vi "Dig.vi"(8 "Error In":errorcluster, 10 "Selection List[]":refnum<vi>[](array[refnum]), 11 "VI In":refnum<vi>) -> (0 "Error Out":errorcluster, 3 "VI Out":refnum<vi>)   [LabVIEW 2017, in "Toolkit VIs.lvlib"]
doc: "A VI script that encloses a selection of code in a Diagram Disable Contional structure, creates a duplicate of the original code to be refactored for the Enabled frame, adds an \"Original\" and \"Refactored\" subdiagram label to each frame, respectively, and adds a bookmark with \"RIP\", the DoD (Date of Death), and grave digger (programmer) as the structure's label.\n\nBy default, today's date is used as the DoD and the application's user name is used for the grave digger."
uses:
  Toolkit VIs.lvlib
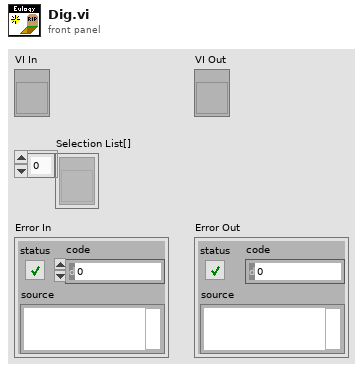
[diagram p1: front panel]
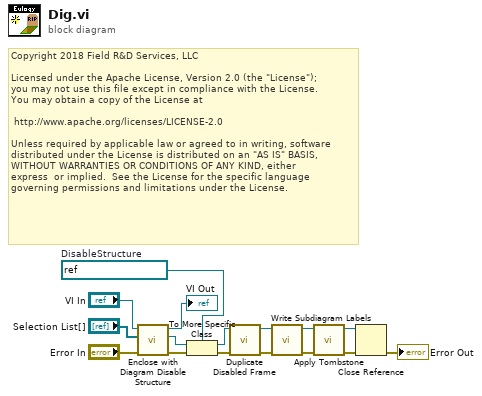
[diagram p0: block diagram]
diagram:
  w15 = refnum<vi> refnum  # DisableStructure
  # "Copyright 2018 Field R&D Services, LLC\n\nLicensed under the Apache License, Version 2.0 (the \"License\");\nyou may not use this file except in compliance with the License.\nYou may obtain a copy of the License at\n\n\thttp://www.apache.org/licenses/LICENSE-2.0\n\nUnless required by applicable law or agreed to in writing, software\ndistributed under the License is distributed on an \"AS IS\" BASIS,\nWITHOUT WARRANTIES OR CONDITIONS OF ANY KIND, either \nexpress  or implied.  See the License for the specific language \ngoverning permissions and limitations under the License."
  n1 = call "Enclose with Diagram Disable Structure.vi"("Error In"="Error In", "Selection List[]"="Selection List[]", "VI In"="VI In") -> ("Error Out"=w9:errorcluster, "Diagram Disable Structure"=w16:refnum<vi>, "VI Out"=→"VI Out":refnum<vi>)  [unwired: 6 in]
  n2 = To More Specific Class(target class=w15, reference=w16, error in=w9) -> (specific class reference=w14:refnum<vi>, error out=w13:errorcluster)
  n3 = call "Duplicate Disabled Frame.vi"("Error In"=w13, "DisableStructure In"=w14) -> ("Error Out"=w12:errorcluster, "DisableStructure Out"=w11:refnum<vi>)  [unwired: 8 in]
  n4 = call "Write Subdiagram Labels.vi"("Error In"=w12, "DisableStructure In"=w11) -> ("Error Out"=w4:errorcluster, "DisableStructure Out"=w10:refnum<vi>)  [unwired: 8 in]
  n5 = call "Apply Tombstone.vi"("Error In"=w4, "Grave In"=w10) -> ("Error Out"=w8:errorcluster, "Grave Out"=w7:refnum<vi>)  [unwired: 8 in]
  n6 = Close Reference(reference=w7, error in (no error)=w8) -> (error out=→"Error Out":errorcluster)
